vi "Create SubPanel.vi"(8 "error in (no error)":errorcluster, 10 "system":refnum<class "multichannel-lockin.lvclass">, 11 "UI.Lockin in":refnum<class "UI.Lockin.lvclass">) -> (0 "error out":errorcluster, 3 "UI.Lockin out":refnum<class "UI.Lockin.lvclass">)   [LabVIEW 2019, in "UI.Lockin.lvclass"]
uses:
  UI.Lockin.lvclass
  C:/Program Files (x86)/National Instruments/LabVIEW 2019/vi.lib/JKI/JKI SMO/SMO/SMO.lvclass
  lockin/multichannel-lockin.lvclass
  UI.Lockin.lvclass/UI.Lockin.ctl
  <vilib>/JKI/JKI SMO/SMO/SMO.lvclass
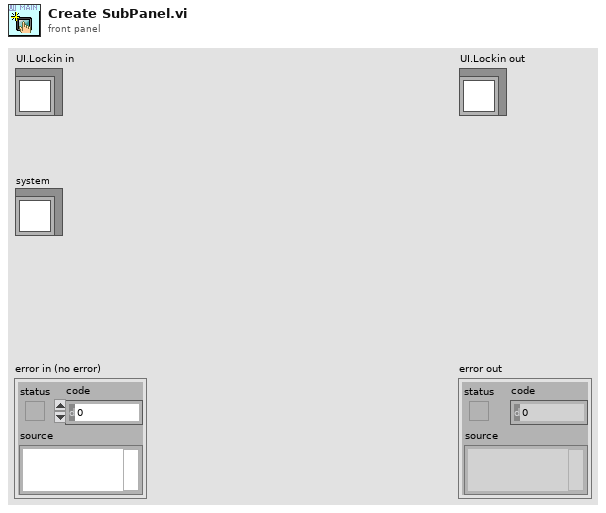
[diagram p1: front panel]
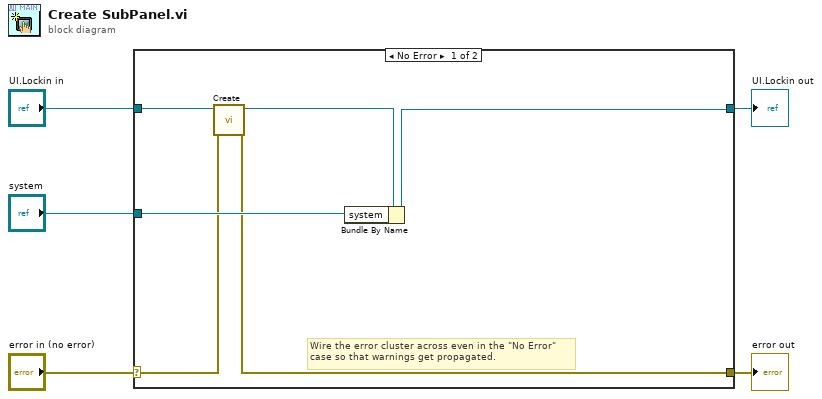
[diagram p0: block diagram]
diagram:
  n1 = case shown="No Error" "error in (no error)" {
    selector: "error in (no error)" -> [w7 w13]
    tunnel: [w6 w13] -> w4
    tunnel: [w9 w12] -> w2
    tunnel: "UI.Lockin in" -> [w11 w12]
    tunnel: "system" -> [w8 _]
    frame No Error {
      # "Wire the error cluster across even in the \"No Error\"\ncase so that warnings get propagated."
      n2 = call <vilib>:"Create.vi"("error in (no error)"=w7, "SMO"=w11) -> ("error out"=w6:errorcluster, "SMO out"=w10:refnum<class "UI.Lockin.lvclass">)  [unwired: 7 in, 1 out]
      n3 = Bundle By Name(cluster=w10, "system"=w8) -> (w9:refnum<class "UI.Lockin.lvclass">)
    }
    frame Error {
    }
  }
  "error out" <- w4
  "UI.Lockin out" <- w2
